vi "Constants.vi"() -> (2 "output cluster":T1)   [LabVIEW 2020]
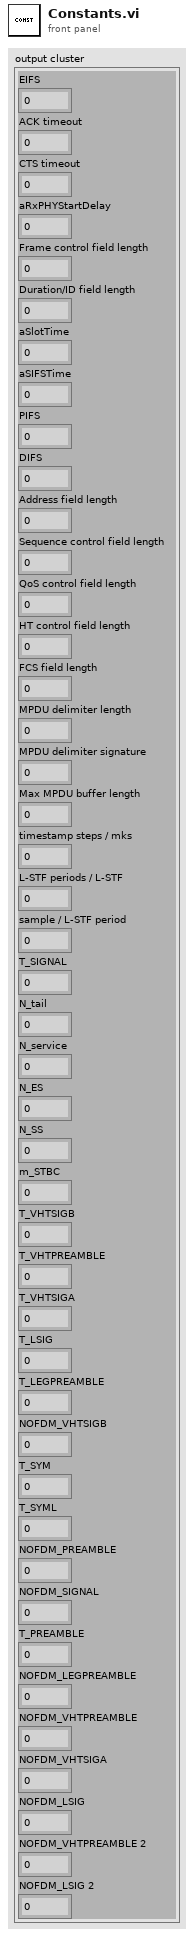
[diagram p1: front panel]
types:
  T1 = cluster{"EIFS":u32, "ACK timeout":u32, "CTS timeout":u32, "aRxPHYStartDelay":u32, "Frame control field length":u16, "Duration/ID field length":u16, "aSlotTime":u32, "aSIFSTime":u32, "PIFS":u32, "DIFS":u32, "Address field length":u16, "Sequence control field length":u16, "QoS control field length":u16, "HT control field length":u16, "FCS field length":u16, "MPDU delimiter length":u16, "MPDU delimiter signature":u16, "Max MPDU buffer length":u16, "timestamp steps / mks":u32, "L-STF periods / L-STF":u8, "sample / L-STF period":u8, "T_SIGNAL":u16, "N_tail":u16, "N_service":u16, "N_ES":u16, "N_SS":u16, "m_STBC":u16, "T_VHTSIGB":u16, "T_VHTPREAMBLE":u16, "T_VHTSIGA":u16, "T_LSIG":u16, "T_LEGPREAMBLE":u16, "NOFDM_VHTSIGB":u16, "T_SYM":u16, "T_SYML":u16, "NOFDM_PREAMBLE":u16, "NOFDM_SIGNAL":u16, "T_PREAMBLE":u16, "NOFDM_LEGPREAMBLE":u16, "NOFDM_VHTPREAMBLE":u16, "NOFDM_VHTSIGA":u16, "NOFDM_LSIG":u16, "NOFDM_VHTPREAMBLE 2":u16, "NOFDM_LSIG 2":u16}
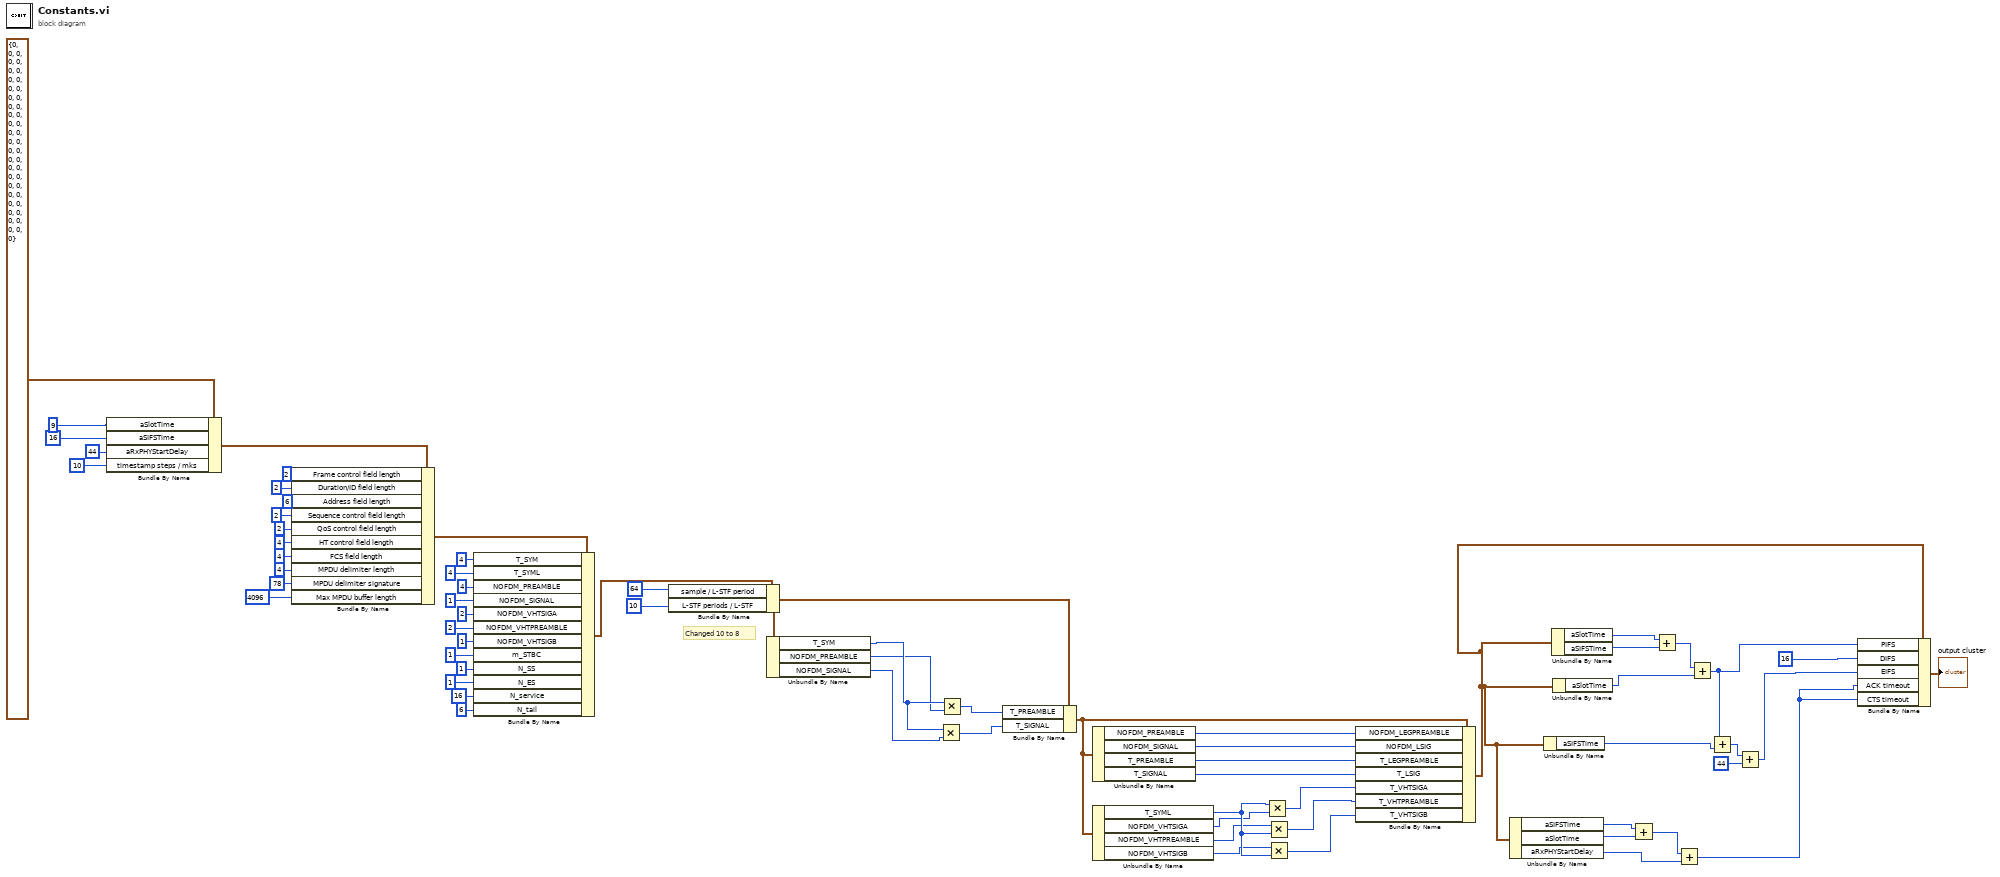
[diagram p0: block diagram]
diagram:
  # "Changed 10 to 8"
  n1 = Bundle By Name(cluster=T1 {"EIFS"=0, "ACK timeout"=0, "CTS timeout"=0, "aRxPHYStartDelay"=0, "Frame control field length"=0, "Duration/ID field length"=0, "aSlotTime"=0, "aSIFSTime"=0, "PIFS"=0, "DIFS"=0, "Address field length"=0, "Sequence control field length"=0, "QoS control field length"=0, "HT control field length"=0, "FCS field length"=0, "MPDU delimiter length"=0, "MPDU delimiter signature"=0, "Max MPDU buffer length"=0, "timestamp steps / mks"=0, "L-STF periods / L-STF"=0, "sample / L-STF period"=0, "T_SIGNAL"=0, "N_tail"=0, "N_service"=0, "N_ES"=0, "N_SS"=0, "m_STBC"=0, "T_VHTSIGB"=0, "T_VHTPREAMBLE"=0, "T_VHTSIGA"=0, "T_LSIG"=0, "T_LEGPREAMBLE"=0, "NOFDM_VHTSIGB"=0, "T_SYM"=0, "T_SYML"=0, "NOFDM_PREAMBLE"=0, "NOFDM_SIGNAL"=0, "T_PREAMBLE"=0, "NOFDM_LEGPREAMBLE"=0, "NOFDM_VHTPREAMBLE"=0, "NOFDM_VHTSIGA"=0, "NOFDM_LSIG"=0, "NOFDM_VHTPREAMBLE 2"=0, "NOFDM_LSIG 2"=0}, "aSlotTime"=u32 9, "aSIFSTime"=u32 16, "aRxPHYStartDelay"=u32 44, "timestamp steps / mks"=u32 10) -> (w62:T1)
  n2 = Bundle By Name(cluster=w62, "Frame control field length"=u16 2, "Duration/ID field length"=u16 2, "Address field length"=u16 6, "Sequence control field length"=u16 2, "QoS control field length"=u16 2, "HT control field length"=u16 4, "FCS field length"=u16 4, "MPDU delimiter length"=u16 4, "MPDU delimiter signature"=u16 78, "Max MPDU buffer length"=u16 4096) -> (w51:T1)
  n3 = Bundle By Name(cluster=w51, "T_SYM"=u16 4, "T_SYML"=u16 4, "NOFDM_PREAMBLE"=u16 4, "NOFDM_SIGNAL"=u16 1, "NOFDM_VHTSIGA"=u16 2, "NOFDM_VHTPREAMBLE"=u16 2, "NOFDM_VHTSIGB"=u16 1, "m_STBC"=u16 1, "N_SS"=u16 1, "N_ES"=u16 1, "N_service"=u16 16, "N_tail"=u16 6) -> (w38:T1)
  n4 = Bundle By Name(cluster=w38, "sample / L-STF period"=u8 64, "L-STF periods / L-STF"=u8 10) -> (w36:T1)
  n5 = Unbundle By Name(w36) -> ("T_SYM"=w35:u16, "NOFDM_PREAMBLE"=w32:u16, "NOFDM_SIGNAL"=w31:u16)
  n6 = Multiply(x=w35, y=w31) -> (x*y=w33:u16)
  n7 = Multiply(x=w35, y=w32) -> (x*y=w34:u16)
  n8 = Bundle By Name(cluster=w36, "T_PREAMBLE"=w34, "T_SIGNAL"=w33) -> (w26:T1)
  n9 = Unbundle By Name(w26) -> ("NOFDM_PREAMBLE"=w27:u16, "NOFDM_SIGNAL"=w28:u16, "T_PREAMBLE"=w29:u16, "T_SIGNAL"=w30:u16)
  n10 = Unbundle By Name(w26) -> ("T_SYML"=w22:u16, "NOFDM_VHTSIGA"=w19:u16, "NOFDM_VHTPREAMBLE"=w20:u16, "NOFDM_VHTSIGB"=w21:u16)
  n11 = Multiply(x=w22, y=w19) -> (x*y=w25:u16)
  n12 = Multiply(x=w20, y=w22) -> (x*y=w24:u16)
  n13 = Multiply(x=w21, y=w22) -> (x*y=w23:u16)
  n14 = Bundle By Name(cluster=w26, "NOFDM_LEGPREAMBLE"=w27, "NOFDM_LSIG"=w28, "T_LEGPREAMBLE"=w29, "T_LSIG"=w30, "T_VHTSIGA"=w25, "T_VHTPREAMBLE"=w24, "T_VHTSIGB"=w23) -> (w14:T1)
  n15 = Unbundle By Name(w14) -> ("aSIFSTime"=w7:u32, "aSlotTime"=w6:u32, "aRxPHYStartDelay"=w4:u32)
  n16 = Unbundle By Name(w14) -> ("aSIFSTime"=w11:u32)
  n17 = Unbundle By Name(w14) -> ("aSlotTime"=w18:u32, "aSIFSTime"=w17:u32)
  n18 = Unbundle By Name(w14) -> ("aSlotTime"=w16:u32)
  n19 = Add(x=w7, y=w6) -> (x+y=w5:u32)
  n20 = Add(x=w18, y=w17) -> (x+y=w15:u32)
  n21 = Add(x=w5, y=w4) -> (x+y=w3:u32)
  n22 = Add(x=w15, y=w16) -> (x+y=w12:u32)
  n23 = Add(x=w12, y=w11) -> (x+y=w10:u32)
  n24 = Add(x=w10, y=u32 44) -> (x+y=w8:u32)
  n25 = Bundle By Name(cluster=w14, "PIFS"=w12, "DIFS"=u32 16, "EIFS"=w8, "ACK timeout"=w3, "CTS timeout"=w3) -> (→"output cluster":T1)
